vi "Lossy Enqueue Element At Opposite End.vi"(8 "error in (no error)":errorcluster, 9 "timeout in ms (-1)":i32=-1, 10 "element":refnum<class "DataObject.lvclass">, 11 "queue in":refnum<queue>) -> (0 "error out":errorcluster, 1 "timed out?":bool, 2 "overflow element":refnum<class "DataObject.lvclass">, 3 "queue out":refnum<queue>)   [LabVIEW 2015, in "QueueOperations.lvlib"]
doc: "https://forums.ni.com/t5/LabVIEW-Idea-Exchange/Lossy-Enqueue-Element-At-Opposite-End/idi-p/3806238"
uses:
  QueueOperations.lvlib
  UndoLibrary/Support VIs/DataClass/DataObject.lvclass
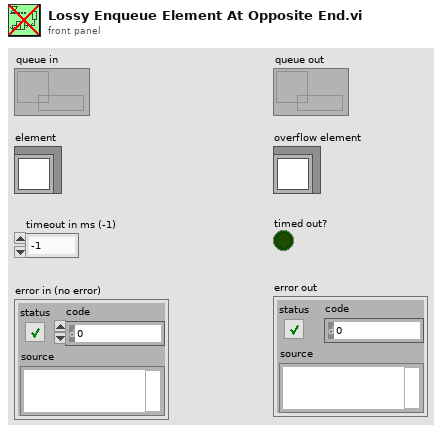
[diagram p1: front panel]
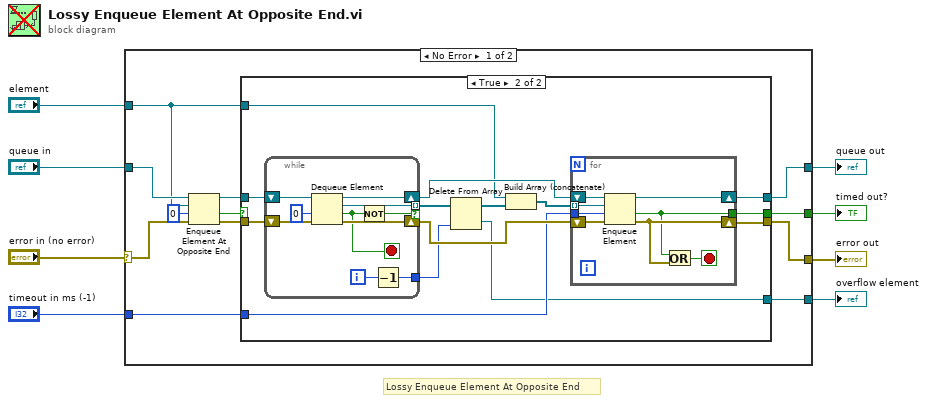
[diagram p0: block diagram]
diagram:
  # "Lossy Enqueue Element At Opposite End"
  n1 = case shown="No Error" "error in (no error)" {
    selector: "error in (no error)" -> [w10 w56]
    tunnel: "timeout in ms (-1)" -> [w16 _]
    tunnel: [w15 _] -> w1
    tunnel: [w14 _] -> w7
    tunnel: [w13 w56] -> w6
    tunnel: [w12 w55] -> w5
    tunnel: "queue in" -> [w11 w55]
    tunnel: "element" -> [w9 _]
    frame No Error {
      n2 = Enqueue Element At Opposite End(queue=w11, element=w9, timeout in ms (-1)=0, error in (no error)=w10) -> (queue out=w17:refnum<queue>, timed out?=w18:bool, error out=w19:errorcluster)
      n3 = case shown="True" w18 {
        tunnel: w19 -> [w21 w35]
        tunnel: w17 -> [w22 w36]
        tunnel: w9 -> [_ w24]
        tunnel: w16 -> [_ w29]
        tunnel: [_ w23] -> w15
        tunnel: [_ w28] -> w14
        tunnel: [w22 w27] -> w12
        tunnel: [w21 w26] -> w13
        frame False {
        }
        frame True {
          n4 = while {
            shift-right: [w52] -> w32
            shift-left: w35 -> [w53]
            tunnel: [w45] -> w34 mode=indexing if=w47
            shift-right: [w51] -> w30
            shift-left: w36 -> [w54]
            tunnel: [w46] -> w25
            i -> [w50]
            stop <- w48 stop-if-true
            n5 = Dequeue Element(queue=w54, timeout in ms (-1)=0, error in (no error)=w53) -> (queue out=w51:refnum<queue>, element=w45:refnum<class "DataObject.lvclass">, timed out?=w48:bool, error out=w52:errorcluster)
            n6 = Not(x=w48) -> (.not. x?=w47:bool)
            n7 = Decrement(x=w50) -> (x-1=w46:i32)
          }
          n8 = Delete From Array(array=w34, index=w25) -> (deleted portion=w23:refnum<class "DataObject.lvclass">, array with subset deleted=w33:refnum<class "DataObject.lvclass">[])  [unwired: 1 in]
          n9 = Build Array (concatenate)(w24, w33) -> (w31:refnum<class "DataObject.lvclass">[])
          n10 = for {
            tunnel: w31 -> [w37] mode=indexing
            tunnel: w29 -> [w42]
            shift-right: [w40] -> w26
            shift-left: w32 -> [w44]
            shift-right: [w39] -> w27
            shift-left: w30 -> [w43]
            tunnel: [w38] -> w28
            stop <- w41 stop-if-true
            n11 = Enqueue Element(queue=w43, element=w37, timeout in ms (-1)=w42, error in (no error)=w44) -> (queue out=w39:refnum<queue>, timed out?=w38:bool, error out=w40:errorcluster)
            n12 = Or(x=w38, y=w40) -> (x .or. y?=w41:bool)
          }
        }
      }
    }
    frame Error {
    }
  }
  "timed out?" <- w7
  "error out" <- w6
  "queue out" <- w5
  "overflow element" <- w1
